vi "Drive with Angle Controller.vi"(9 "Angle Increment":dbl, 11 "Straight Speed":dbl) -> (2 "Right Motor Value":dbl, 3 "Left Motor Value":dbl)   [LabVIEW 2016]
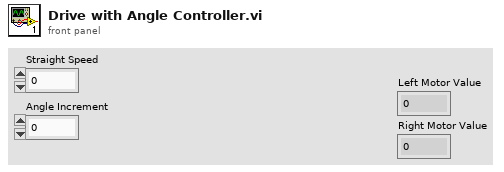
[diagram p1: front panel]
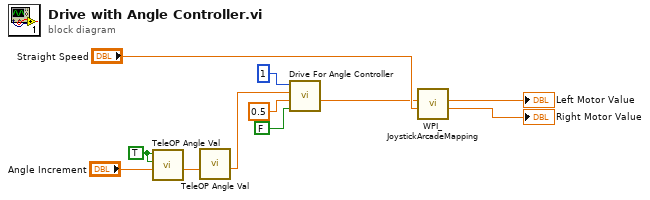
[diagram p0: block diagram]
diagram:
  w2 = TRUE ("Write")
  n1 = call "TeleOP Angle Val.vi"("TeleOP Angle (in)"="Angle Increment", "Add"=w2, "Write"=w2) -> ("TeleOP Angle (out)"=w5:dbl)  [unwired: 8 in]
  n2 = call "TeleOP Angle Val.vi"("TeleOP Angle (in)"=w5) -> ("TeleOP Angle (out)"=w4:dbl)  [unwired: 10 in]
  n3 = call "Drive For Angle Controller.vi"("Vision"=FALSE, "Speed"=0.5, "Yaw"=w4, "Iterations"=1) -> ("Right Setpoint"=w1:dbl)  [unwired: 5 in, 2 out]
  n4 = call <vilib>:"WPI_JoystickArcadeMapping.vi"("Y axis value"="Straight Speed", "X axis value"=w1) -> ("Right Motor Value"=→"Right Motor Value":dbl, "Left Motor Value"=→"Left Motor Value":dbl)  [unwired: 8 in]
